vi "Read Inputs from system.vi"(8 "error in":errorcluster, 11 "GPIC ScaleAndLimit runtime in":refnum<class "GPIC ScaleAndLimit runtime.lvclass">) -> (0 "error out":errorcluster, 2 "Inputs from system":T1, 3 "GPIC ScaleAndLimit runtime out":refnum<class "GPIC ScaleAndLimit runtime.lvclass">)   [LabVIEW 2015, in "GPIC ScaleAndLimit runtime.lvclass"]
uses:
  GPIC ScaleAndLimit runtime.lvclass
  configuration/input data indices.ctl
  GPIC ScaleAndLimit runtime.lvclass/GPIC ScaleAndLimit runtime.ctl
  configuration/GPIC ScaleAndLimit configuration.lvclass
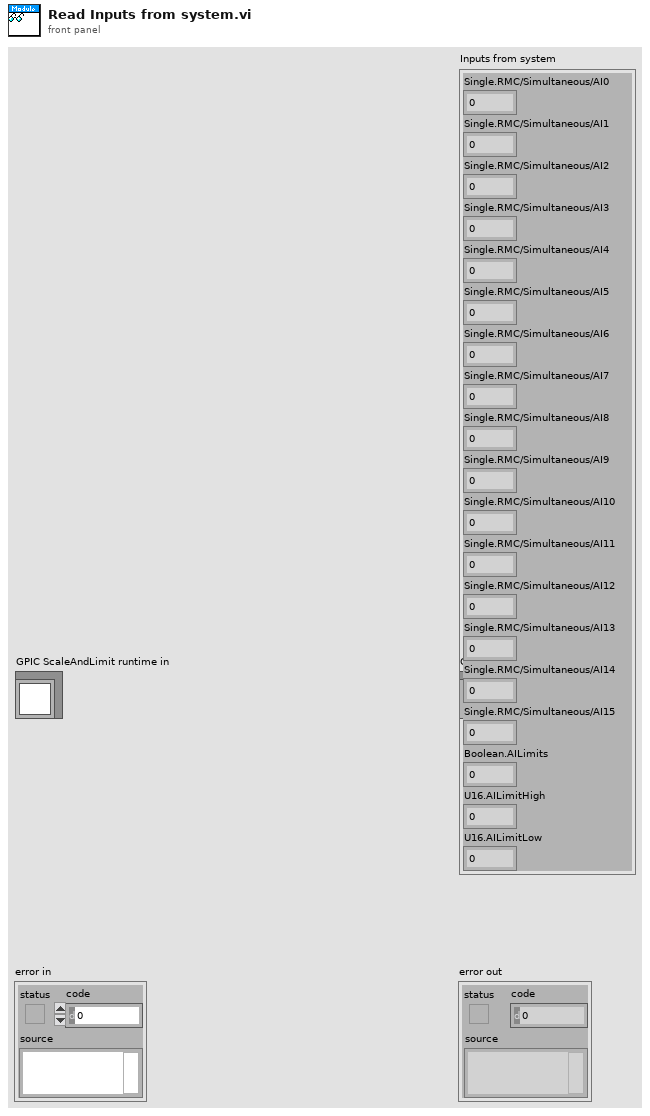
[diagram p1: front panel]
types:
  T1 = typedef "GPIC ScaleAndLimit configuration.lvclass/input data indices.ctl" = cluster{"Single.RMC/Simultaneous/AI0":i32, "Single.RMC/Simultaneous/AI1":i32, "Single.RMC/Simultaneous/AI2":i32, "Single.RMC/Simultaneous/AI3":i32, "Single.RMC/Simultaneous/AI4":i32, "Single.RMC/Simultaneous/AI5":i32, "Single.RMC/Simultaneous/AI6":i32, "Single.RMC/Simultaneous/AI7":i32, "Single.RMC/Simultaneous/AI8":i32, "Single.RMC/Simultaneous/AI9":i32, "Single.RMC/Simultaneous/AI10":i32, "Single.RMC/Simultaneous/AI11":i32, "Single.RMC/Simultaneous/AI12":i32, "Single.RMC/Simultaneous/AI13":i32, "Single.RMC/Simultaneous/AI14":i32, "Single.RMC/Simultaneous/AI15":i32, "Boolean.AILimits":i32, "U16.AILimitHigh":i32, "U16.AILimitLow":i32}
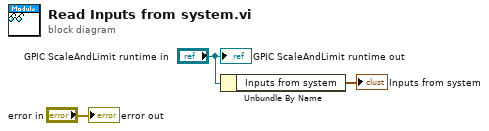
[diagram p0: block diagram]
diagram:
  n1 = Unbundle By Name("GPIC ScaleAndLimit runtime in") -> ("Inputs from system"=→"Inputs from system":T1)
  "error out" <- "error in"
  "GPIC ScaleAndLimit runtime out" <- "GPIC ScaleAndLimit runtime in"
